vi "UpdateIndicators.vi"(7 "VI in":refnum<vi>, 8 "error in (no error)":errorcluster, 9 "Channel Name":string[](array[string]), 10 "Control Index":i32[](array[numeric]), 11 "WorkspaceManager in":T1) -> (0 "error out":errorcluster, 3 ".NET Refnum out":T1)   [LabVIEW 2017]
uses:
  <vilib>/NI Veristand/Execution/Workspace/WorkspaceAPI.ctl
  NationalInstruments.VeriStand.ClientAPI
  <vilib>/NI Veristand/Execution/Workspace/NI VeriStand - Get Multiple Channel Values.vi
  <vilib>/NI Veristand/Execution/Workspace/NI_VS Workspace ExecutionAPI.lvlib
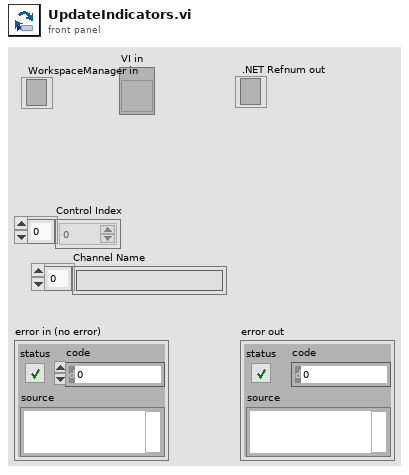
[diagram p1: front panel]
types:
  T1 = typedef "NI_VS Workspace ExecutionAPI.lvlib/WorkspaceAPI.ctl" = refnum<k24>
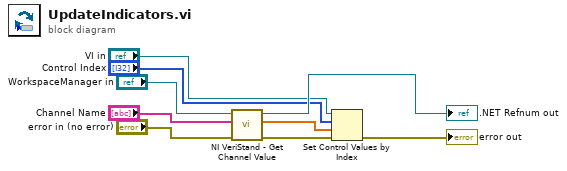
[diagram p0: block diagram]
diagram:
  n1 = call-poly <vilib>:"NI VeriStand - Get Channel Value.vi"("error in (no error)"="error in (no error)", "Channels"="Channel Name", "WorkspaceManager in"="WorkspaceManager in") -> ("error out"=w8:errorcluster, "Values"=w6:dbl[], "WorkspaceManager out"=→".NET Refnum out":T1)  [unwired: 6 in]
  n2 = Set Control Values by Index(0:"VI in", 1:"Control Index", 2:w6, 3:w8) -> (11:→"error out":errorcluster)
